vi "ControlInterface.vi"() -> ()   [LabVIEW 2016]
uses:
  Classes/CAlex2-Display/CAlex2_Display.lvclass
  D:/JinXin/LabVIEW.git/CAlex2-Controller-treadmill/Classes/SerialChain/SerialChain.lvclass
  D:/JinXin/LabVIEW.git/CAlex2-Controller-treadmill/Classes/CAlex2/CAlex2.lvclass
  Classes/ForceField/TypeDef/FF_Gains.ctl
  Classes/CAlex2/TypeDef/LowerBodyDim.ctl
  Classes/MotorControl/TypeDef/ControllerMode.ctl
  Classes/MotorControl/MotorControl.lvclass
  Classes/CAlex2/CAlex2.lvclass
  Classes/SerialChain/SerialChain.lvclass
  Classes/ForceField/ForceField.lvclass
  <vilib>/GoldZinc Software/auzn custom VIs/CustomVI.lvlib
panel:
  in  "FF Disp Type":enum16{"FF: XYZ", "FF: NTD"}(ring)
  in  "Motor Mode":T1={"Idle"=FALSE, "Pre"=FALSE, "Pre-Value"=7, "PID"=FALSE} {"Pre-Value" items=["7N"=7, "10N"=10, "15N"=15, "20N"=20]}
  out "ViconConnected":bool
  in  "ResetIMU":bool
  in  "Vicon":bool
  in  "Extra Wt":cluster{"Thigh (lb)":dbl, "Shank (lb)":dbl}
  in  "UpdateFF":bool
  in  "XZ":bool
  in  "YZ":bool
  in  "XY":bool
  out "R_Hill":u32(colorbox)
  out "R_Ball":u32(colorbox)
  out "R_Toe":u32(colorbox)
  out "L_Hill":u32(colorbox)
  out "L_Ball":u32(colorbox)
  out "L_Toe":u32(colorbox)
  in  "Status 8":bool
  out "Waveform Chart 8":cluster{"[0]":dbl, "[1]":dbl}(graph)
  in  "Cuff Location":T2={"Hip Wd (m)"=0.42, "Hip Ht (m)"=0.2, "ThighDist (in)"=1.5, "ThighToKnee"=0.1, "Hip Fwd (m)"=-0.02, "ShankToKnee"=0.1}
  in  "Force Field":bool
  in  "LegWeight":bool
  in  "CuffWeight":bool
  out "Normal Force Shape":cluster{dbl[], dbl[]}[](graph)
  in  "File Name":string
  out "Record Time":dbl format="%.2f"
  in  "Leg Property":T3={"Thigh"=0.42, "Shank"=0.42, "ShankWt"=0.0, "ThighWt"=0.0, "Hip"=0.32}
  in  "Gains":T4
  in  "Reset":bool
  in  "Stop RT":bool
  in  "Status 7":bool
  in  "Status 6":bool
  in  "Status 5":bool
  in  "Status 4":bool
  in  "Status 3":bool
  in  "Status 2":bool
  in  "Status 1":bool
  out "Waveform Chart 7":cluster{"[0]":dbl, "[1]":dbl}(graph)
  out "Waveform Chart 6":cluster{"[0]":dbl, "[1]":dbl}(graph)
  out "Waveform Chart 5":cluster{"[0]":dbl, "[1]":dbl}(graph)
  out "Waveform Chart 4":cluster{"[0]":dbl, "[1]":dbl}(graph)
  out "Waveform Chart 3":cluster{"[0]":dbl, "[1]":dbl}(graph)
  out "Waveform Chart 2":cluster{"[0]":dbl, "[1]":dbl}(graph)
  out "Waveform Chart 1":cluster{"[0]":dbl, "[1]":dbl}(graph)
  in  "ZeroPosition":bool
  in  "Force Field Type":u8(ring)=1 items=["Ankle Traj", "Ankle Traj 2", "No FF", "Ankle Traj Old"]
  in  "Record Data?":bool
  out "Planned Tensions":dbl[](array[numeric]) format="%.2f"
  out "Motor Command":dbl[](array[numeric]) format="%.5f"
  out "Ankle Center":dbl[](array[numeric]) format="%.4f"
  out "Force Field":dbl[](array[numeric]) format="%.2f"
  out "Joint Angles":dbl[](array[numeric]) format="%.1f"
  in  "TareIMU":bool
  in  "Leg Position":refnum<k7>(container)
  # "C-ALEX Control Interface V2 \nDeveloped by Xin Jin, ROAR Laboratory, Columbia University"
  # "Leg Pose"
  # "Status Monitor"
  # "Data Record"
  # "Subject Information"
  # "Foot Switches"
  # "Force Field"
  # "Control Panel"
  # "Motor Mode"
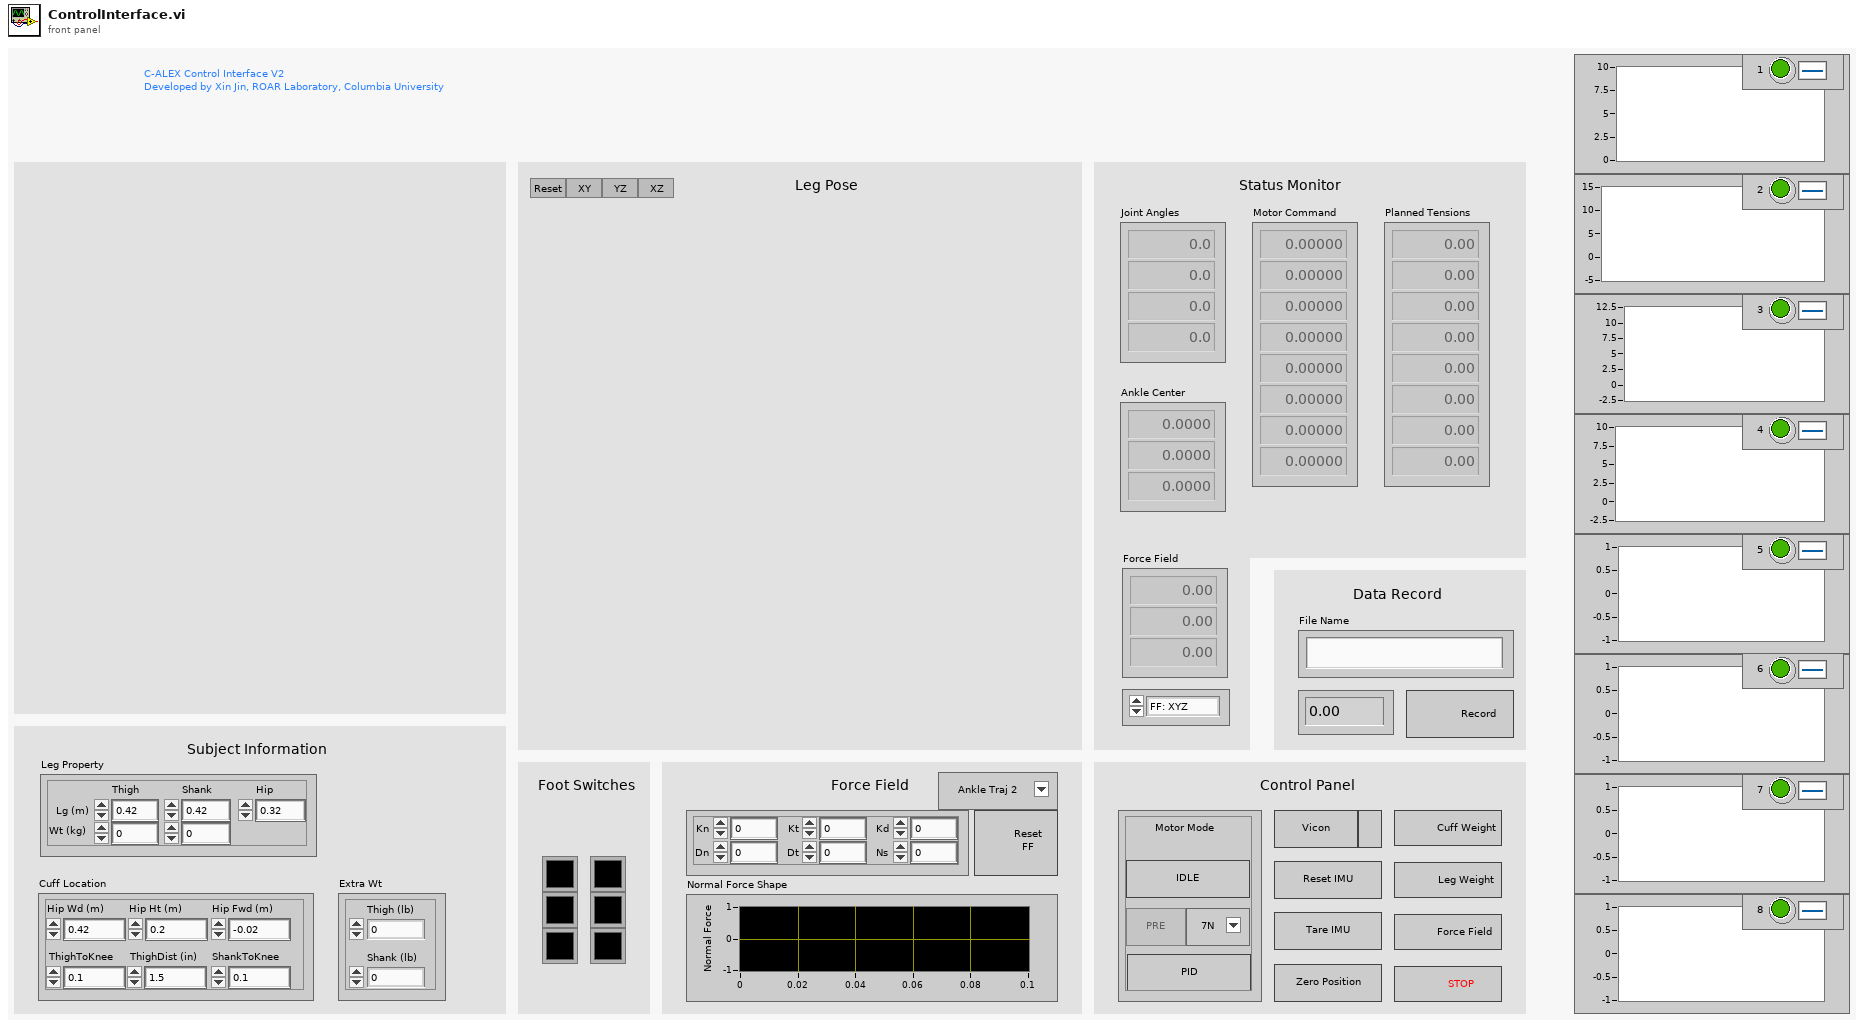
[diagram p1: front panel]
types:
  T1 = cluster{"Idle":bool, "Pre":bool, "Pre-Value":u8, "PID":bool}
  T2 = cluster{"Hip Wd (m)":dbl, "Hip Ht (m)":dbl, "ThighDist (in)":dbl, "ThighToKnee":dbl, "Hip Fwd (m)":dbl, "ShankToKnee":dbl}
  T3 = cluster{"Thigh":dbl, "Shank":dbl, "ShankWt":dbl, "ThighWt":dbl, "Hip":dbl}
  T4 = cluster{"Kn":dbl, "Dn":dbl, "Kt":dbl, "Dt":dbl, "Kd":dbl, "Ns":dbl}
  T5 = cluster{"AxisLabel":string[], "AxisMax":dbl[], "AxisMin":dbl[]}
  T6 = typedef "ForceField.lvclass/FF_Gains.ctl" = cluster{"Kn":dbl, "Dn":dbl, "Kt":dbl, "Dt":dbl, "Kd":dbl, "Ns":dbl}
  T7 = typedef "CAlex2.lvclass/LowerBodyDim.ctl" = cluster{"BodyDim":cluster{"ThighLt (m)":dbl, "ShankLt (m)":dbl, "HipWd (m)":dbl}, "BodyWt":cluster{"Thigh (kg)":dbl, "Shank (kg)":dbl}, "Cuff Loc":cluster{"HipCuffWd (m)":dbl, "HipCuffHt (m)":dbl, "HipFwdShift (m)":dbl, "ThighToKnee (m)":dbl, "ThighCuffDist (m)":dbl, "ShankToKnee (m)":dbl}}
  T8 = typedef "MotorControl.lvclass/ControllerMode.ctl" = enum16{"Idle", "FF", "PID"}
  T9 = enum8{"Enabled", "Disabled", "Disabled and Grayed Out"}
  T10 = cluster{"Input":enum16{"Fr:Cable", "Fr:Motor", "Fr:Sensor"}, "Output":enum16{"To:Cable", "To:Motor", "To:Sensor"}}
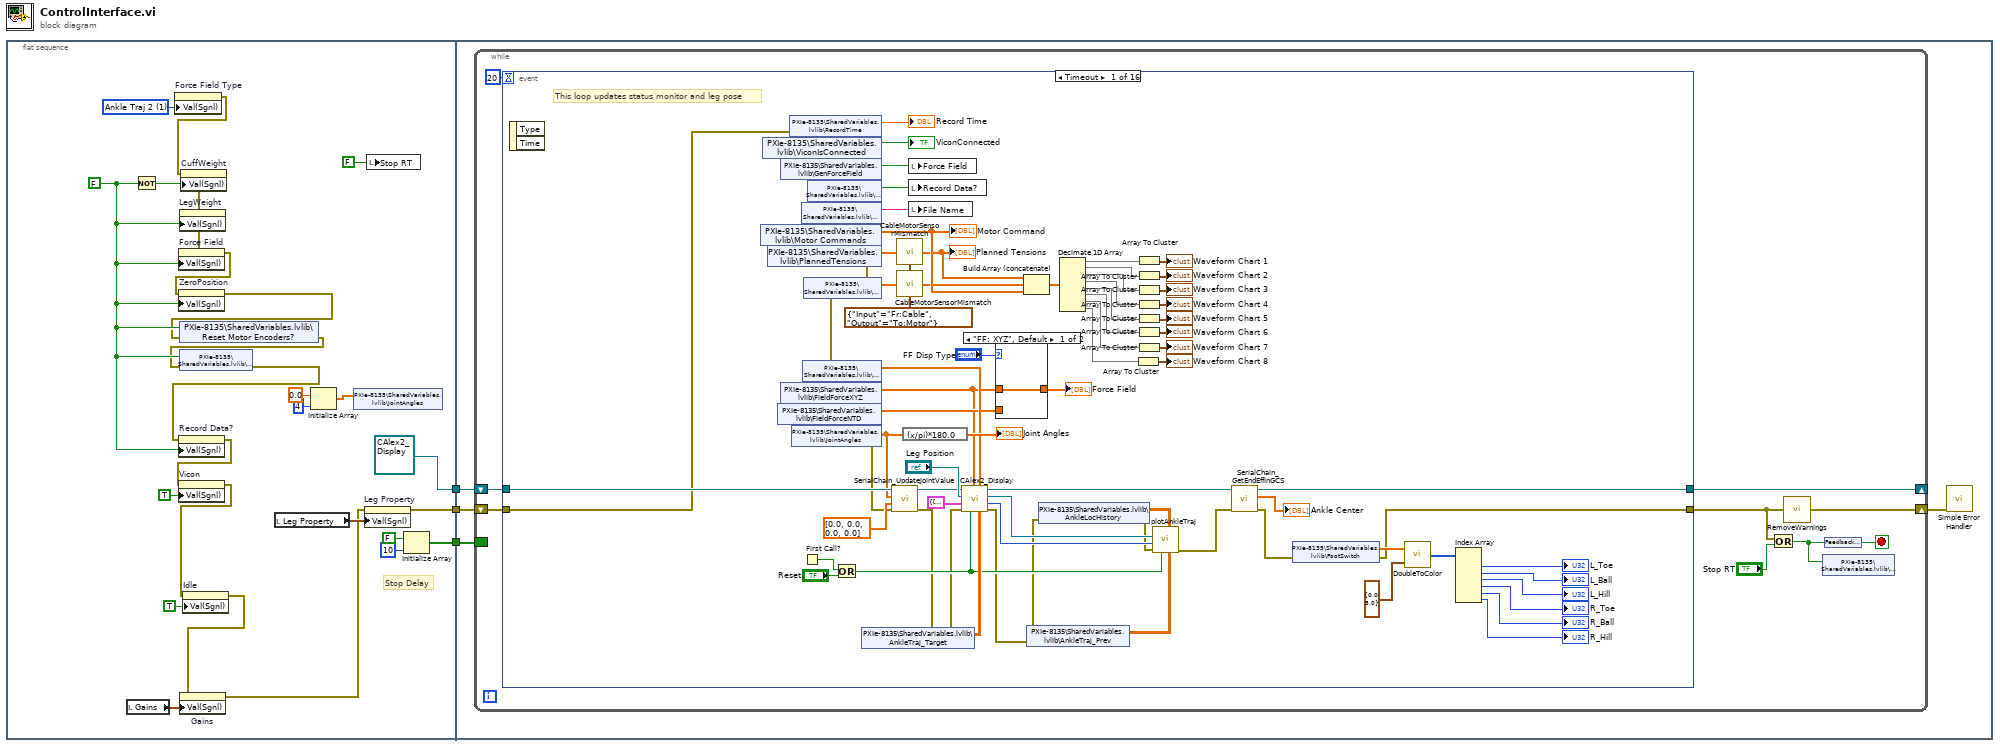
[diagram p0: block diagram]
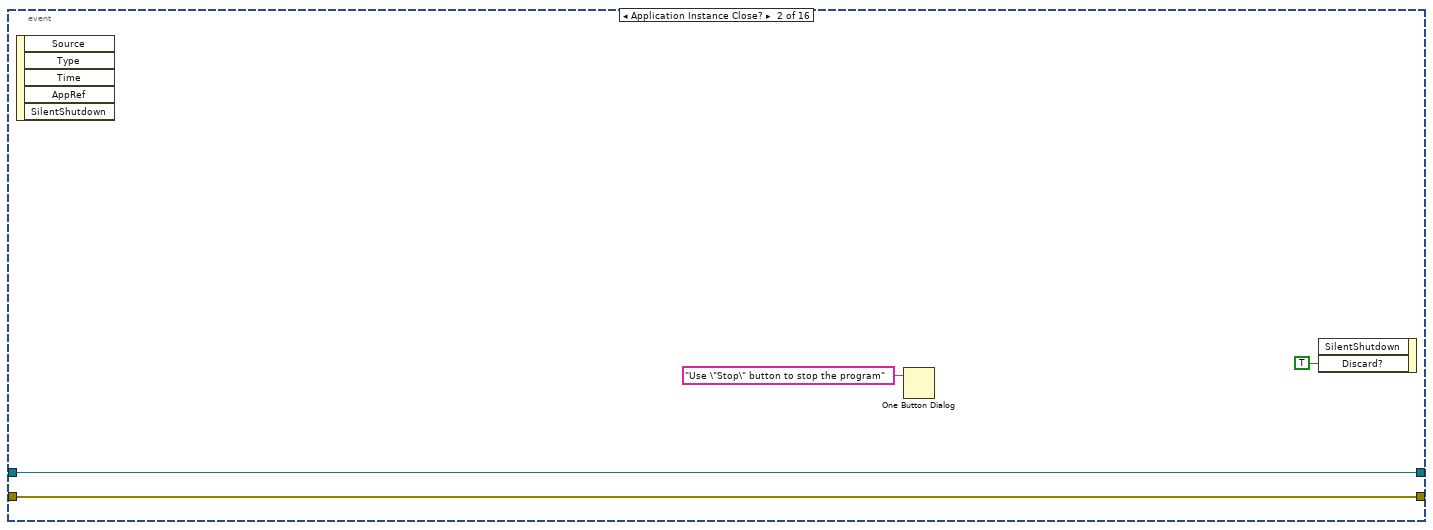
[diagram p3: hidden frame]
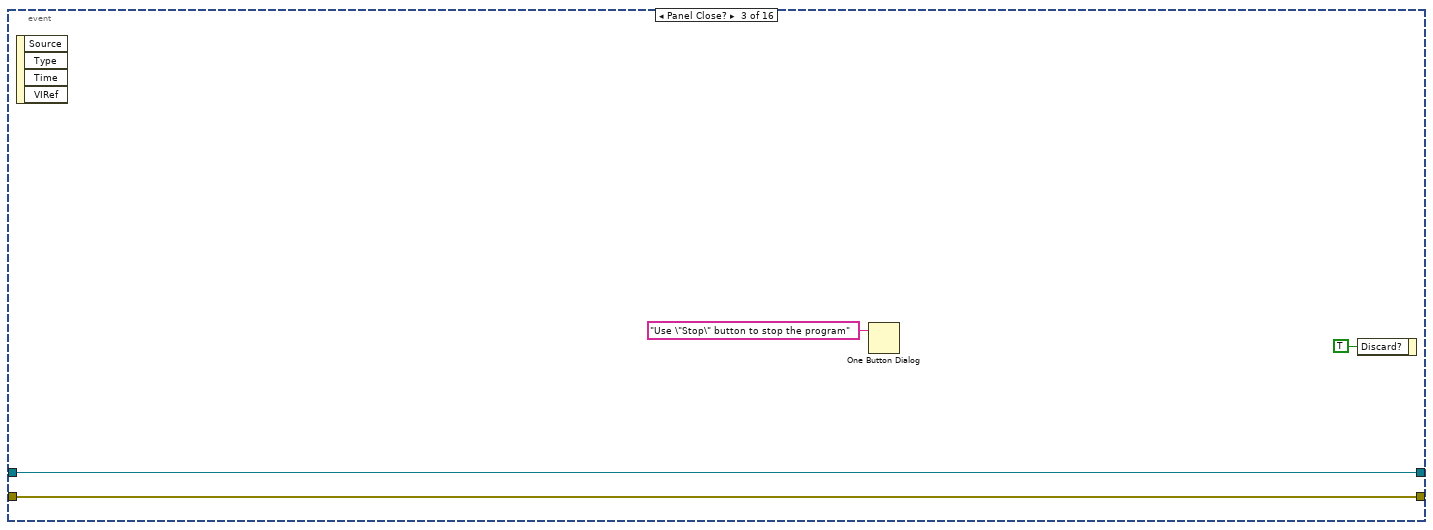
[diagram p4: hidden frame]
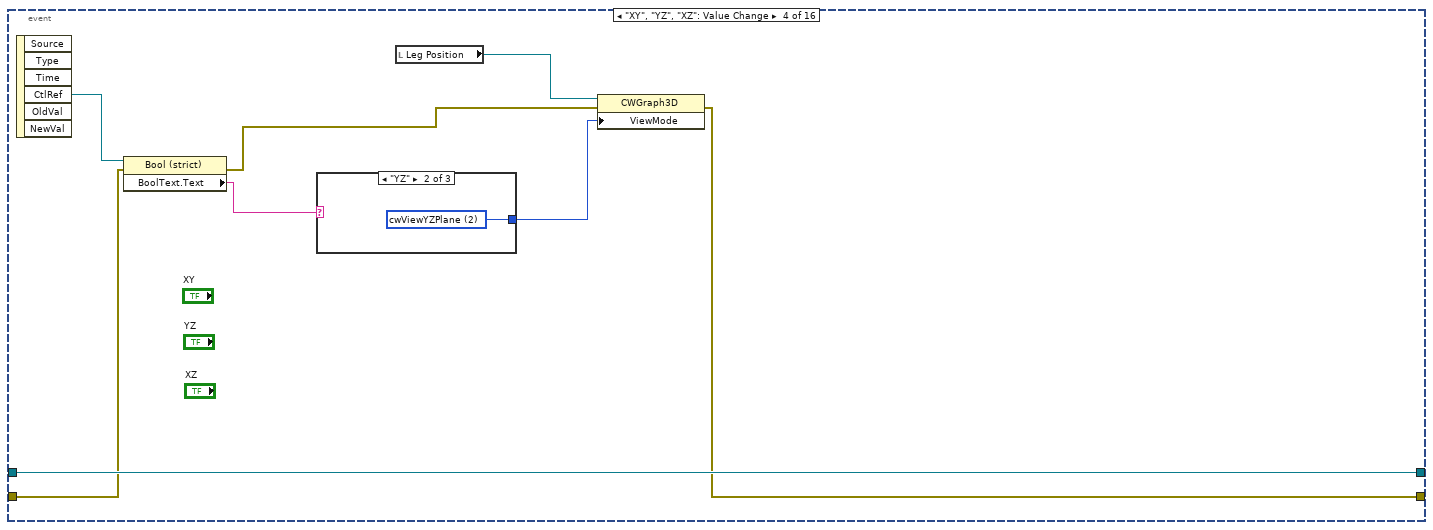
[diagram p5: hidden frame]
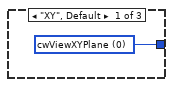
[diagram p6: hidden frame]
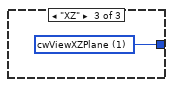
[diagram p7: hidden frame]
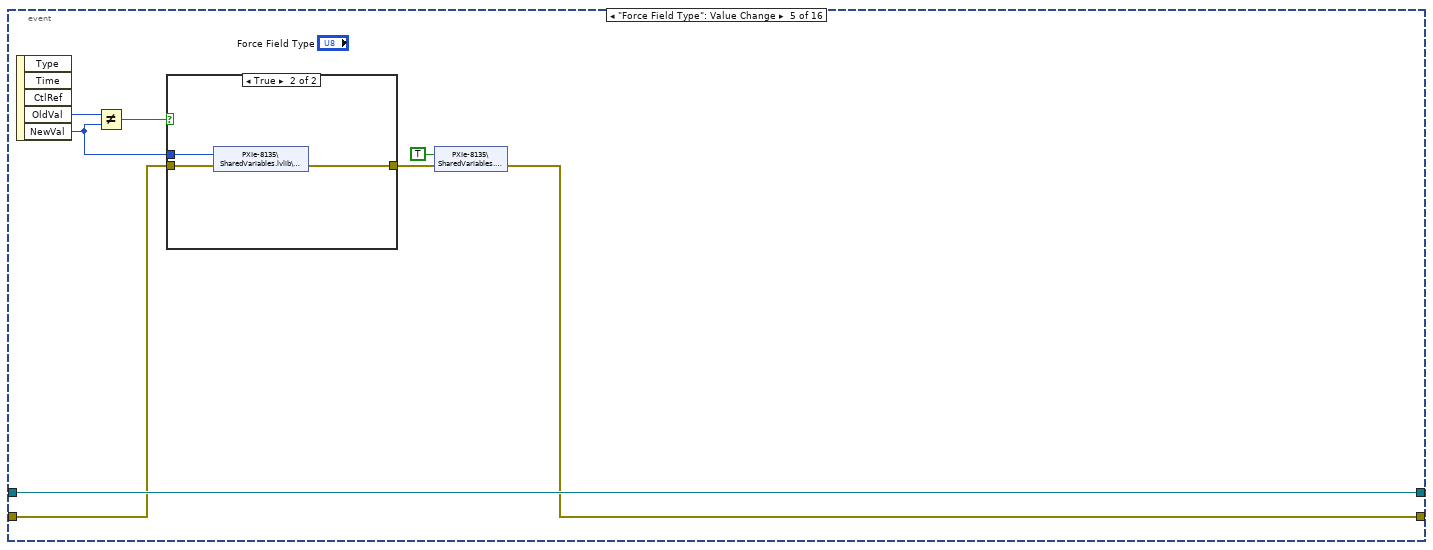
[diagram p8: hidden frame]
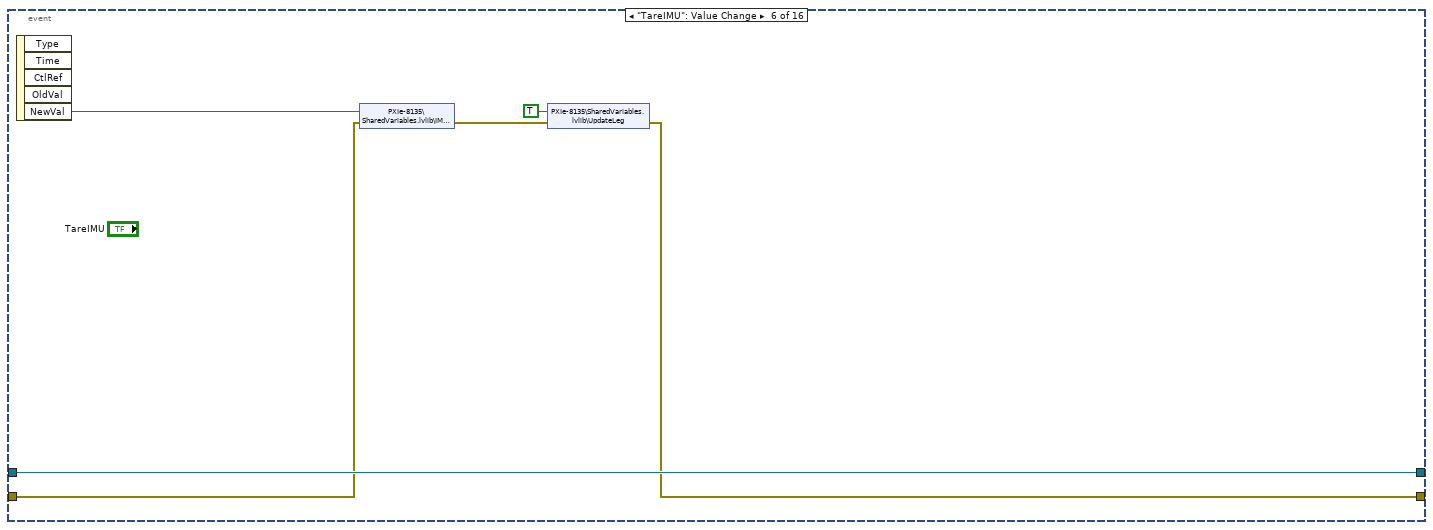
[diagram p10: hidden frame]
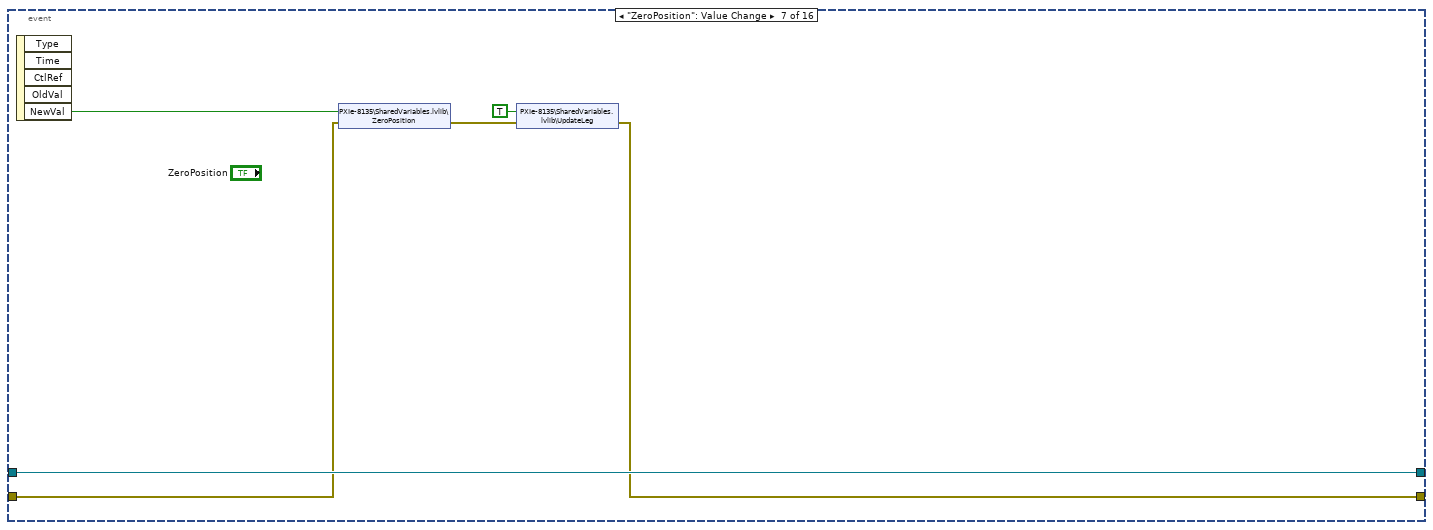
[diagram p11: hidden frame]
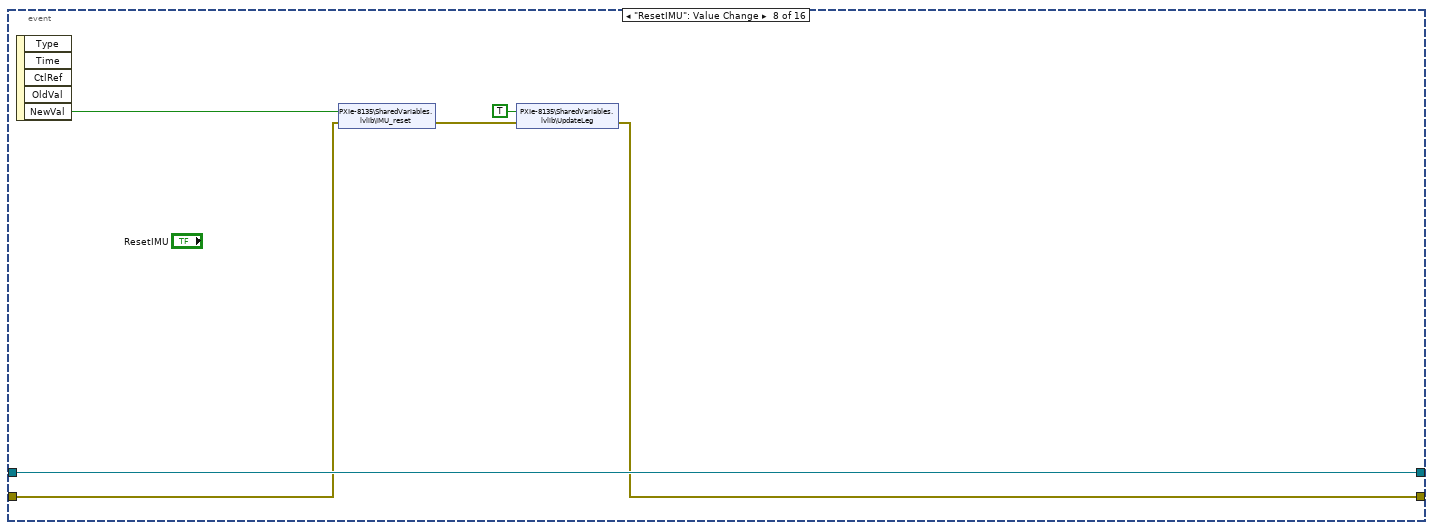
[diagram p12: hidden frame]
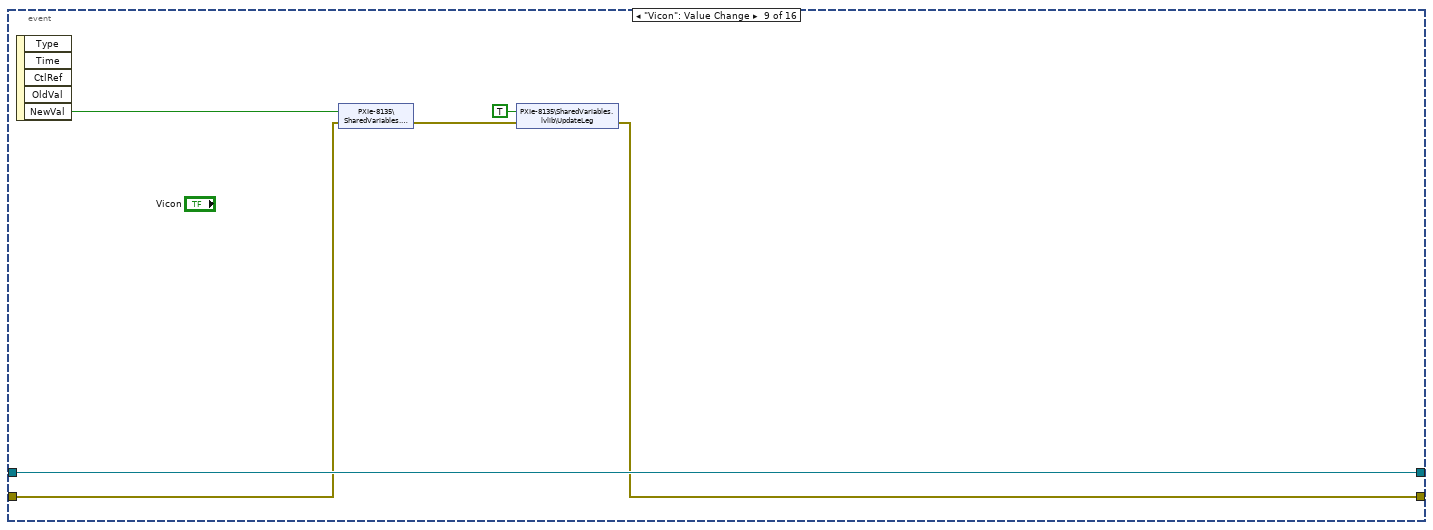
[diagram p13: hidden frame]
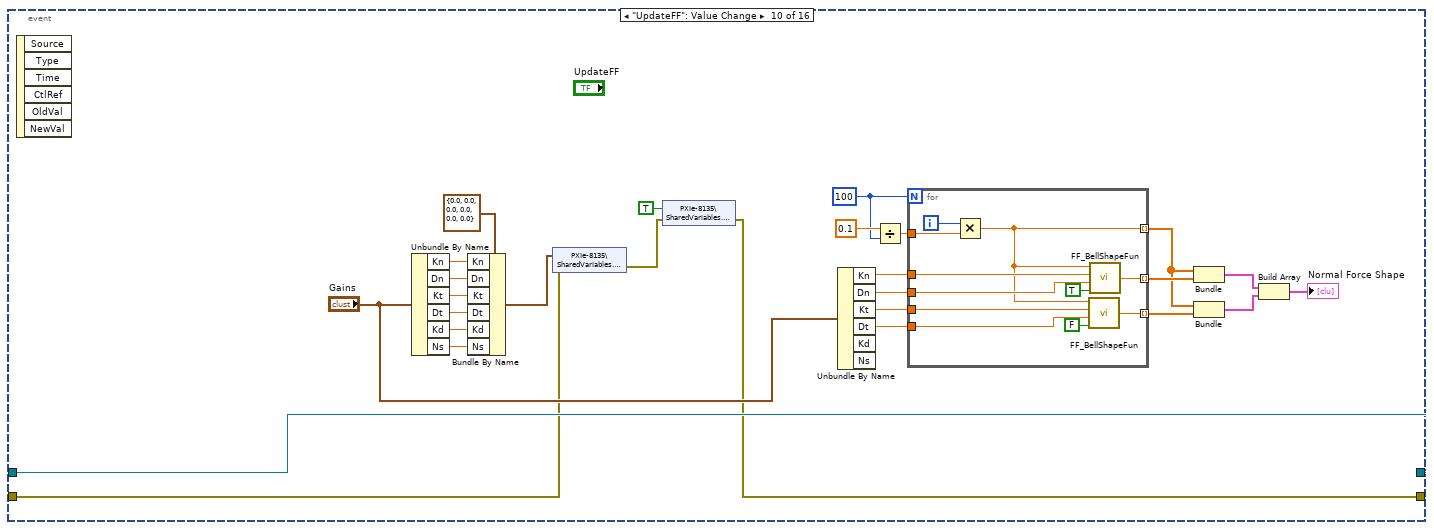
[diagram p14: hidden frame]
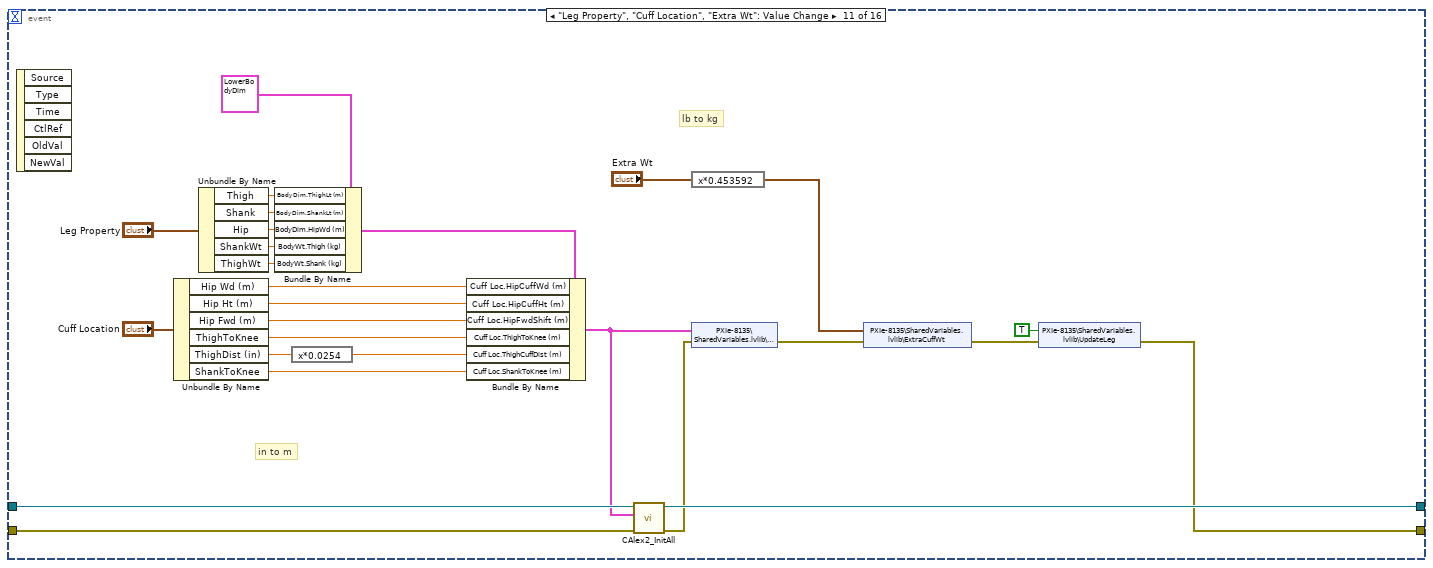
[diagram p15: hidden frame]
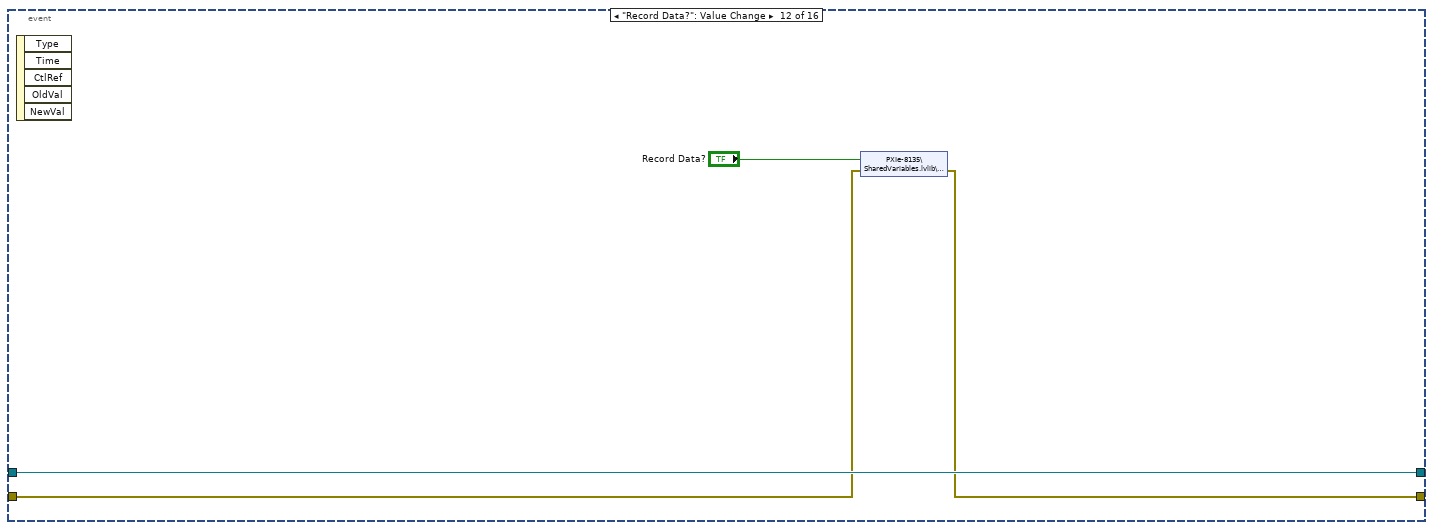
[diagram p16: hidden frame]
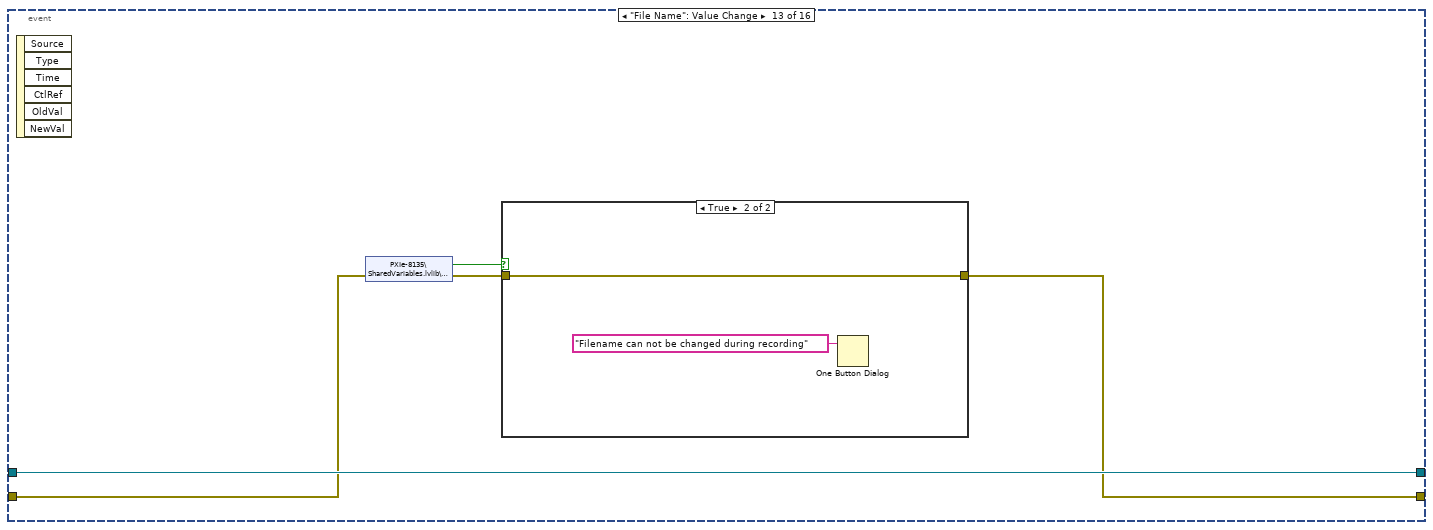
[diagram p17: hidden frame]
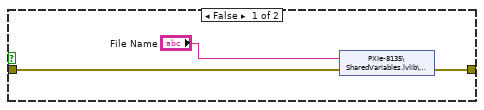
[diagram p18: hidden frame]
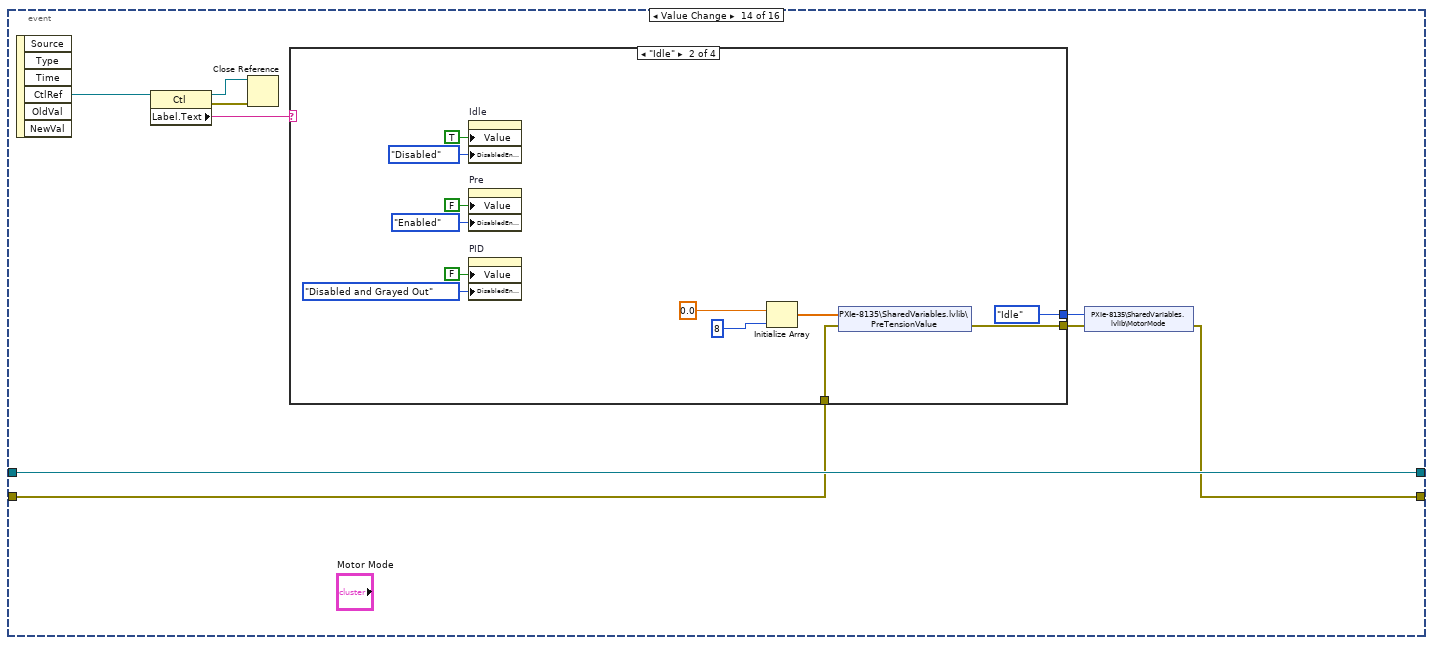
[diagram p19: hidden frame]
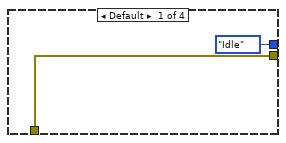
[diagram p20: hidden frame]
diagram:
  n1 = flat-sequence {
    tunnel: [w28] -> w3
    tunnel: [refnum<class "CAlex2_Display.lvclass"> refnum ("CAlex2")] -> w2
    tunnel: [w22] -> w1
    tunnel: w3 -> [w32]
    tunnel: w2 -> [w34]
    tunnel: w1 -> [w33]
    frame #0 {
      w17 = u8 1 items=["Ankle Traj", "Ankle Traj 2", "No FF", "Ankle Traj Old"] ("Force Field Type")
      w10 = FALSE ("Es SH Center?")
      # "Stop Delay"
      n2 = local read "Gains"() -> (w27:T4)
      n3 = Not(x=w10) -> (.not. x?=w11:bool)
      n4 = property on="Force Field Type" class="Ring (strict)"("Val(Sgnl)"=w17) -> (error out=w5:errorcluster)  [unwired: 2 in, 1 out]
      n5 = property on="CuffWeight" class="Bool (strict)"(error in=w5, "Val(Sgnl)"=w11) -> (error out=w13:errorcluster)  [unwired: 1 in, 1 out]
      n6 = property on="LegWeight" class="Bool (strict)"(error in=w13, "Val(Sgnl)"=w10) -> (error out=w12:errorcluster)  [unwired: 1 in, 1 out]
      n7 = property on="Force Field" class="Bool (strict)"(error in=w12, "Val(Sgnl)"=w10) -> (error out=w9:errorcluster)  [unwired: 1 in, 1 out]
      n8 = property on="ZeroPosition" class="Bool (strict)"(error in=w9, "Val(Sgnl)"=w10) -> (error out=w8:errorcluster)  [unwired: 1 in, 1 out]
      n9 = shared-variable "PXIe-8135\\SharedVariables.lvlib\\Reset Motor Encoders?"(w10, error in=w8) -> (error out=w7:errorcluster)
      n10 = shared-variable "PXIe-8135\\SharedVariables.lvlib\\Stop RT"(w10, error in=w7) -> (error out=w4:errorcluster)
      n11 = property on="Record Data?" class="Bool (strict)"(error in=w4, "Val(Sgnl)"=w10) -> (error out=w15:errorcluster)  [unwired: 1 in, 1 out]
      n12 = property on="Vicon" class="Bool (strict)"(error in=w15, "Val(Sgnl)"=TRUE ("Value (Signaling)")) -> (error out=w16:errorcluster)  [unwired: 1 in, 1 out]
      n13 = property on="Idle" class="Bool (strict)"(error in=w16, "Val(Sgnl)"=TRUE ("Value")) -> (error out=w6:errorcluster)  [unwired: 1 in, 1 out]
      n14 = property on="Gains" class="Clust (strict)"(error in=w6, "Val(Sgnl)"=w27) -> (error out=w26:errorcluster)  [unwired: 1 in, 1 out]
      n15 = local read "Leg Property"() -> (w29:T3)
      n16 = Initialize Array(0.0 ("element"), 4 ("dimension size")) -> (w20:dbl[])
      n17 = shared-variable "PXIe-8135\\SharedVariables.lvlib\\JointAngles"(w20) -> ()  [unwired: 1 in, 1 out]
      n18 = property on="Leg Property" class="Clust (strict)"(error in=w26, "Val(Sgnl)"=w29) -> (error out=w28:errorcluster)  [unwired: 1 in, 1 out]
      n19 = local write "Stop RT"(FALSE ("Es SH Center?")) -> ()
      n20 = Initialize Array(FALSE, 10 ("dimension size")) -> (w22:bool[])
    }
    frame #1 {
      n21 = while {
        shift-right: [w41] -> _
        shift-left: w34 -> [w42]
        border: w33 -> [_]
        shift-right: [w38] -> w31
        shift-left: w32 -> [w39]
        stop <- w40 stop-if-true
        n22 = event shown="[0] Timeout" {
          selector: _ -> [_ _ _ _ _ _ _ _ _ _ _ _ _ _ _ _]
          dyn-events: _ -> [_ _ _ _ _ _ _ _ _ _ _ _ _ _ _ _]
          timeout: 20 -> [_ _ _ _ _ _ _ _ _ _ _ _ _ _ _ _]
          tunnel: [w70 w130 w134 w139 w148 w160 w167 w173 w179 w182 w241 w248 w254 w263 w306 w314] -> w37
          tunnel: w42 -> [w106 w129 w133 w142 w150 w163 w169 w175 w181 w208 w246 w250 w255 w269 w312 w324]
          tunnel: w39 -> [w44 w130 w134 w136 w147 w161 w168 w174 w180 w183 w244 w247 w253 w261 w305 w315]
          tunnel: [w104 w129 w133 w142 w150 w163 w169 w175 w181 w208 w245 w250 w255 w269 w312 w324] -> w41
          event Timeout {
            w71 = T10 {"Input"=enum."Fr:Cable", "Output"=enum."To:Motor"} ("Conversion")
            # "This loop updates status monitor and leg pose"
            n23 = event-data() -> ()  [unwired: 1 in, 2 out]
            n24 = shared-variable "PXIe-8135\\SharedVariables.lvlib\\RecordTime"(error in=w44) -> (→"Record Time":dbl, error out=w76:errorcluster)
            n25 = shared-variable "PXIe-8135\\SharedVariables.lvlib\\ViconIsConnected"(error in=w76) -> (→"ViconConnected":bool, error out=w52:errorcluster)
            n26 = shared-variable "PXIe-8135\\SharedVariables.lvlib\\GenForceField"(error in=w52) -> (w61:bool, error out=w62:errorcluster)
            n27 = First Call?() -> (First Call?: T/F=w107:bool)
            n28 = shared-variable "PXIe-8135\\SharedVariables.lvlib\\Record?"(error in=w62) -> (w59:bool, error out=w60:errorcluster)
            n29 = shared-variable "PXIe-8135\\SharedVariables.lvlib\\FileName"(error in=w60) -> (w51:string, error out=w50:errorcluster)
            n30 = shared-variable "PXIe-8135\\SharedVariables.lvlib\\Motor Commands"(error in=w50) -> (w100:dbl[], error out=w124:errorcluster)
            "Motor Command" <- w100
            n31 = shared-variable "PXIe-8135\\SharedVariables.lvlib\\PlannedTensions"(error in=w124) -> (w73:dbl[], error out=w101:errorcluster)
            n32 = shared-variable "PXIe-8135\\SharedVariables.lvlib\\Tensions"(error in=w101) -> (w75:dbl[], error out=w45:errorcluster)
            n33 = shared-variable "PXIe-8135\\SharedVariables.lvlib\\ClosestPt"(error in=w45) -> (w92:dbl[], error out=w69:errorcluster)
            n34 = shared-variable "PXIe-8135\\SharedVariables.lvlib\\FieldForceXYZ"(error in=w69) -> (w55:dbl[], error out=w53:errorcluster)
            n35 = shared-variable "PXIe-8135\\SharedVariables.lvlib\\FieldForceNTD"(error in=w53) -> (w56:dbl[], error out=w47:errorcluster)
            n36 = shared-variable "PXIe-8135\\SharedVariables.lvlib\\JointAngles"(error in=w47) -> (w102:dbl[], error out=w46:errorcluster)
            n37 = Or(x=w107, y="Reset") -> (x .or. y?=w89:bool)
            n38 = call "SerialChain_UpdateJointValue.vi"("error in (no error)"=w46, "JointSpeed (rad/s | m/s)"=dbl[] [0.0, 0.0, 0.0, 0.0] ("JointSpeed (rad)"), "JointAngle (rad | m)"=w102, "SerialChain in"=w106) -> ("error out"=w48:errorcluster, "SerialChain out"=w96:refnum<class "CAlex2_Display.lvclass">)  [unwired: 6 in]
            n39 = shared-variable "PXIe-8135\\SharedVariables.lvlib\\AnkleTraj_Target"(error in=w48) -> (w93:dbl[][], error out=w68:errorcluster)
            n40 = call "CableMotorSensorMismatch.vi"("Conversion"=w71, "Input"=w73) -> ("Output"=w72:dbl[])  [unwired: 2 in]
            "Planned Tensions" <- w72
            n41 = call "CableMotorSensorMismatch.vi"("Conversion"=w71, "Input"=w75) -> ("Output"=w74:dbl[])  [unwired: 2 in]
            n42 = expression code="(x/pi)*180.0" ("radians to degrees")(w102) -> (→"Joint Angles":dbl[])
            n43 = local write "Force Field"(w61) -> ()
            n44 = local write "Record Data?"(w59) -> ()
            n45 = local write "File Name"(w51) -> ()
            n46 = call "CAlex2_Display.vi"("AnkleTraj_Target"=w93, "ClosePt"=w92, "Init?"=w89, "Field Force"=w55, "error in (no error)"=w68, "AxisSetting"=T5 {"AxisLabel"=["x ", "y", "z "], "AxisMax"=[0.75, 0.3, 0.8], "AxisMin"=[-0.75, -1.2, -0.7]}, "3D graph in"="Leg Position", "CLX2 in"=w96) -> ("error out"=w67:errorcluster, "LastPlotNum"=w90:i32, "3D graph out"=w91:refnum<k7>, "CLX2 out"=w98:refnum<class "CAlex2_Display.lvclass">)
            n47 = case shown="\"FF: XYZ\", Default" "FF Disp Type" {
              tunnel: w56 -> [_ w126]
              tunnel: w55 -> [w125 _]
              tunnel: [w125 w126] -> w54
              frame "FF: XYZ", Default {
              }
              frame "FF: NTD" {
              }
            }
            "Force Field" <- w54
            n48 = Build Array (concatenate)(w72, w74, w100) -> (w99:dbl[])
            n49 = shared-variable "PXIe-8135\\SharedVariables.lvlib\\AnkleTraj_Prev"(error in=w67) -> (w88:dbl[][], error out=w64:errorcluster)
            n50 = shared-variable "PXIe-8135\\SharedVariables.lvlib\\AnkleLocHistory"(error in=w64) -> (w65:dbl[][], error out=w63:errorcluster)
            n51 = Decimate 1D Array(w99) -> (w117:dbl[], w116:dbl[], w122:dbl[], w121:dbl[], w120:dbl[], w119:dbl[], w118:dbl[], w49:dbl[])
            n52 = Array To Cluster(array=w49) -> (cluster=→"Waveform Chart 8":cluster{"[0]":dbl, "[1]":dbl})
            n53 = Array To Cluster(array=w117) -> (cluster=→"Waveform Chart 1":cluster{"[0]":dbl, "[1]":dbl})
            n54 = Array To Cluster(array=w116) -> (cluster=→"Waveform Chart 2":cluster{"[0]":dbl, "[1]":dbl})
            n55 = Array To Cluster(array=w122) -> (cluster=→"Waveform Chart 3":cluster{"[0]":dbl, "[1]":dbl})
            n56 = Array To Cluster(array=w121) -> (cluster=→"Waveform Chart 4":cluster{"[0]":dbl, "[1]":dbl})
            n57 = Array To Cluster(array=w120) -> (cluster=→"Waveform Chart 5":cluster{"[0]":dbl, "[1]":dbl})
            n58 = Array To Cluster(array=w119) -> (cluster=→"Waveform Chart 6":cluster{"[0]":dbl, "[1]":dbl})
            n59 = Array To Cluster(array=w118) -> (cluster=→"Waveform Chart 7":cluster{"[0]":dbl, "[1]":dbl})
            n60 = call "plotAnkleTraj.vi"("AnkleTraj_Prev"=w88, "AnkleTraj_history"=w65, "Init?"=w89, "error in (no error)"=w63, "PreviousPlotNum"=w90, "3D graph in"=w91) -> ("error out"=w66:errorcluster)  [unwired: 3 in, 2 out]
            n61 = call "SerialChain_GetEndEffInGCS.vi"("error in (no error)"=w66, "SerialChain in"=w98) -> ("error out"=w58:errorcluster, "Pendeff(GCS)"=→"Ankle Center":dbl[], "SerialChain out"=w104:refnum<class "CAlex2_Display.lvclass">)  [unwired: 5 in, 2 out]
            n62 = shared-variable "PXIe-8135\\SharedVariables.lvlib\\FootSwitch"(error in=w58) -> (w87:dbl[], error out=w70:errorcluster)
            n63 = call <vilib>:"DoubleToColor.vi"("Value Range"=cluster{"ValueMin":dbl, "ValueMax":dbl} {"ValueMin"=0.0, "ValueMax"=5.0}, "Data"=w87) -> ("Colors"=w85:u32[])  [unwired: 1 in]
            n64 = Index Array(array=w85) -> (element #1=→"L_Toe":u32, element #2=→"L_Ball":u32, element #3=→"L_Hill":u32, element #4=→"R_Toe":u32, element #5=→"R_Ball":u32, element #6=→"R_Hill":u32)  [unwired: 6 in]
          }
          event Application Instance Close? {
            n65 = event-data() -> ()  [unwired: 1 in, 5 out]
            n66 = One Button Dialog(message="Use \"Stop\" button to stop the program") -> ()  [unwired: 1 in, 1 out]
            n67 = event-data("Discard?"=TRUE) -> ()  [unwired: 2 in, 1 out]
          }
          event Panel Close? {
            n68 = event-data() -> ()  [unwired: 1 in, 4 out]
            n69 = One Button Dialog(message="Use \"Stop\" button to stop the program") -> ()  [unwired: 1 in, 1 out]
            n70 = event-data("Discard?"=TRUE) -> ()  [unwired: 1 in, 1 out]
          }
          event "XY", "YZ", "XZ": Value Change {
            n71 = event-data() -> ("CtlRef"=w138:refnum<vi>)  [unwired: 1 in, 5 out]
            n72 = property class="Bool (strict)"(reference=w138, error in=w136) -> (error out=w137:errorcluster, "BoolText.Text"=w135:string)  [unwired: 1 out]
            n73 = case shown="\"YZ\"" w135 {
              tunnel: [w143 w144 w145] -> w140
              frame "XY", Default {
                w143 = 0 items=["cwViewXYPlane", "cwViewXZPlane", "cwViewYZPlane", "cwViewUserDefined"] ("ViewMode")
              }
              frame "YZ" {
                w144 = 2 items=["cwViewXYPlane", "cwViewXZPlane", "cwViewYZPlane", "cwViewUserDefined"] ("ViewMode")
              }
              frame "XZ" {
                w145 = 1 items=["cwViewXYPlane", "cwViewXZPlane", "cwViewYZPlane", "cwViewUserDefined"] ("ViewMode")
              }
            }
            n74 = local read "Leg Position"() -> (w141:refnum<k7>)
            n75 = property class="CWGraph3D"(reference=w141, error in=w137, "ViewMode"=w140) -> (error out=w139:errorcluster)  [unwired: 1 out]
          }
          event "Force Field Type": Value Change {
            n76 = event-data() -> ("OldVal"=w153:u8, "NewVal"=w151:u8)  [unwired: 1 in, 3 out]
            n77 = Not Equal?(x=w153, y=w151) -> (x != y?=w152:bool)
            n78 = case shown="True" w152 {
              tunnel: w151 -> [_ w157]
              tunnel: [w154 w155] -> w149
              tunnel: w147 -> [w154 w156]
              frame False {
              }
              frame True {
                n79 = shared-variable "PXIe-8135\\SharedVariables.lvlib\\PathType"(w157, error in=w156) -> (error out=w155:errorcluster)
              }
            }
            n80 = shared-variable "PXIe-8135\\SharedVariables.lvlib\\FFRst"(TRUE ("UpdateArm"), error in=w149) -> (error out=w148:errorcluster)
          }
          event "TareIMU": Value Change {
            n81 = event-data() -> ("NewVal"=w162:bool)  [unwired: 1 in, 4 out]
            n82 = shared-variable "PXIe-8135\\SharedVariables.lvlib\\IMU_Tare"(w162, error in=w161) -> (error out=w158:errorcluster)
            n83 = shared-variable "PXIe-8135\\SharedVariables.lvlib\\UpdateLeg"(TRUE ("UpdateArm"), error in=w158) -> (error out=w160:errorcluster)
          }
          event "ZeroPosition": Value Change {
            n84 = event-data() -> ("NewVal"=w166:bool)  [unwired: 1 in, 4 out]
            n85 = shared-variable "PXIe-8135\\SharedVariables.lvlib\\ZeroPosition"(w166, error in=w168) -> (error out=w164:errorcluster)
            n86 = shared-variable "PXIe-8135\\SharedVariables.lvlib\\UpdateLeg"(TRUE ("UpdateArm"), error in=w164) -> (error out=w167:errorcluster)
          }
          event "ResetIMU": Value Change {
            n87 = event-data() -> ("NewVal"=w172:bool)  [unwired: 1 in, 4 out]
            n88 = shared-variable "PXIe-8135\\SharedVariables.lvlib\\IMU_reset"(w172, error in=w174) -> (error out=w170:errorcluster)
            n89 = shared-variable "PXIe-8135\\SharedVariables.lvlib\\UpdateLeg"(TRUE ("UpdateArm"), error in=w170) -> (error out=w173:errorcluster)
          }
          event "Vicon": Value Change {
            n90 = event-data() -> ("NewVal"=w178:bool)  [unwired: 1 in, 4 out]
            n91 = shared-variable "PXIe-8135\\SharedVariables.lvlib\\Vicon"(w178, error in=w180) -> (error out=w176:errorcluster)
            n92 = shared-variable "PXIe-8135\\SharedVariables.lvlib\\UpdateLeg"(TRUE ("UpdateArm"), error in=w176) -> (error out=w179:errorcluster)
          }
          event "UpdateFF": Value Change {
            w193 = 100
            n93 = event-data() -> ()  [unwired: 1 in, 6 out]
            n94 = Unbundle By Name("Gains") -> ("Kn"=w207:dbl, "Dn"=w205:dbl, "Kt"=w204:dbl, "Dt"=w203:dbl, "Kd"=w202:dbl, "Ns"=w201:dbl)
            n95 = Bundle By Name(cluster=T6 {"Kn"=0.0, "Dn"=0.0, "Kt"=0.0, "Dt"=0.0, "Kd"=0.0, "Ns"=0.0} ("Gains"), "Kn"=w207, "Dn"=w205, "Kt"=w204, "Dt"=w203, "Kd"=w202, "Ns"=w201) -> (w200:T6)
            n96 = shared-variable "PXIe-8135\\SharedVariables.lvlib\\Gains"(w200, error in=w183) -> (error out=w184:errorcluster)
            n97 = shared-variable "PXIe-8135\\SharedVariables.lvlib\\FFRst"(TRUE ("UpdateArm"), error in=w184) -> (error out=w182:errorcluster)
            n98 = Unbundle By Name("Gains") -> ("Kn"=w198:dbl, "Dn"=w197:dbl, "Kt"=w196:dbl, "Dt"=w195:dbl)  [unwired: 2 out]
            n99 = Divide(x=0.1, y=w193) -> (x/y=w192:dbl)
            n100 = for {
              N: w193 -> [_]
              tunnel: w198 -> [w219]
              tunnel: w197 -> [w218]
              tunnel: w196 -> [w217]
              tunnel: w195 -> [w216]
              tunnel: w192 -> [w212]
              tunnel: [w211] -> w189 mode=indexing
              tunnel: [w210] -> w190 mode=indexing
              tunnel: [w209] -> w191 mode=indexing
              i -> [w213]
              n101 = Multiply(x=w213, y=w212) -> (x*y=w211:dbl)
              n102 = call "FF_BellShapeFun.vi"("Invert(F)"=FALSE, "(r)adius"=w216, "(A)mplitude"=w217, "x"=w211) -> ("y"=w209:dbl)  [unwired: 2 in]
              n103 = call "FF_BellShapeFun.vi"("Invert(F)"=TRUE ("Invert"), "(r)adius"=w218, "(A)mplitude"=w219, "x"=w211) -> ("y"=w210:dbl)  [unwired: 2 in]
            }
            n104 = Bundle(w189, w190) -> (w187:cluster{dbl[], dbl[]})  [unwired: 1 in]
            n105 = Bundle(w189, w191) -> (w188:cluster{dbl[], dbl[]})  [unwired: 1 in]
            n106 = Build Array(w187, w188) -> (→"Normal Force Shape":cluster{dbl[], dbl[]}[])
          }
          event "Leg Property", "Cuff Location", "Extra Wt": Value Change {
            # "in to m"
            # "lb to kg"
            n107 = event-data() -> ()  [unwired: 1 in, 6 out]
            n108 = Unbundle By Name("Cuff Location") -> ("Hip Wd (m)"=w230:dbl, "Hip Ht (m)"=w229:dbl, "Hip Fwd (m)"=w228:dbl, "ThighToKnee"=w227:dbl, "ThighDist (in)"=w226:dbl, "ShankToKnee"=w225:dbl)
            n109 = Unbundle By Name("Leg Property") -> ("Thigh"=w236:dbl, "Shank"=w237:dbl, "Hip"=w238:dbl, "ShankWt"=w239:dbl, "ThighWt"=w240:dbl)
            n110 = Bundle By Name(cluster=T7 {"BodyDim"={"ThighLt (m)"=0.4, "ShankLt (m)"=0.41, "HipWd (m)"=0.32}, "BodyWt"={"Thigh (kg)"=0.0, "Shank (kg)"=0.0}, "Cuff Loc"={"HipCuffWd (m)"=0.4, "HipCuffHt (m)"=0.1, "HipFwdShift (m)"=0.0, "ThighToKnee (m)"=0.25, "ThighCuffDist (m)"=0.0, "ShankToKnee (m)"=0.15}} ("LegProperties"), "BodyDim.ThighLt (m)"=w236, "BodyDim.ShankLt (m)"=w237, "BodyDim.HipWd (m)"=w238, "BodyWt.Thigh (kg)"=w239, "BodyWt.Shank (kg)"=w240) -> (w233:T7)
            n111 = expression code="x*0.0254"(w226) -> (w220:dbl)
            n112 = Bundle By Name(cluster=w233, "Cuff Loc.HipCuffWd (m)"=w230, "Cuff Loc.HipCuffHt (m)"=w229, "Cuff Loc.HipFwdShift (m)"=w228, "Cuff Loc.ThighToKnee (m)"=w227, "Cuff Loc.ThighCuffDist (m)"=w220, "Cuff Loc.ShankToKnee (m)"=w225) -> (w232:T7)
            n113 = call "CAlex2_InitAll.vi"("error in (no error)"=w244, "LegProperties"=w232, "CAlex2 in"=w246) -> ("error out"=w243:errorcluster, "CAlex2 out"=w245:refnum<class "CAlex2_Display.lvclass">)  [unwired: 7 in]
            n114 = expression code="x*0.453592"("Extra Wt") -> (w221:cluster{"Thigh (lb)":dbl, "Shank (lb)":dbl})
            n115 = shared-variable "PXIe-8135\\SharedVariables.lvlib\\LegDim"(w232, error in=w243) -> (error out=w224:errorcluster)
            n116 = shared-variable "PXIe-8135\\SharedVariables.lvlib\\ExtraCuffWt"(w221, error in=w224) -> (error out=w223:errorcluster)
            n117 = shared-variable "PXIe-8135\\SharedVariables.lvlib\\UpdateLeg"(TRUE ("UpdateArm"), error in=w223) -> (error out=w241:errorcluster)
          }
          event "Record Data?": Value Change {
            n118 = event-data() -> ()  [unwired: 1 in, 5 out]
            n119 = shared-variable "PXIe-8135\\SharedVariables.lvlib\\Record?"("Record Data?", error in=w247) -> (error out=w248:errorcluster)
          }
          event "File Name": Value Change {
            n120 = event-data() -> ()  [unwired: 1 in, 6 out]
            n121 = shared-variable "PXIe-8135\\SharedVariables.lvlib\\Record?"(error in=w253) -> (w251:bool, error out=w252:errorcluster)
            n122 = case shown="True" w251 {
              tunnel: [w258 w260] -> w254
              tunnel: w252 -> [w257 w260]
              frame False {
                n123 = shared-variable "PXIe-8135\\SharedVariables.lvlib\\FileName"("File Name", error in=w257) -> (error out=w258:errorcluster)
              }
              frame True {
                n124 = One Button Dialog(message="Filename can not be changed during recording") -> ()  [unwired: 1 in, 1 out]
              }
            }
          }
          event "Motor Mode.Idle", "Motor Mode.Pre", "Motor Mode.PID", "Motor Mode.Pre-Value": Value Change {
            n125 = event-data() -> ("CtlRef"=w267:refnum<vi>)  [unwired: 1 in, 5 out]
            n126 = property class="Ctl"(reference=w267) -> (reference out=w264:refnum<vi>, error out=w265:errorcluster, "Label.Text"=w266:string)  [unwired: 1 in]
            n127 = Close Reference(reference=w264, error in (no error)=w265) -> ()  [unwired: 1 out]
            n128 = case shown="\"Idle\"" w266 {
              tunnel: [ControllerMode."Idle" ("MotorMode") ControllerMode."Idle" ("MotorMode") ControllerMode."FF" ("MotorMode") ControllerMode."PID" ("MotorMode")] -> w268
              tunnel: [w270 w273 w285 w297] -> w262
              tunnel: w261 -> [w270 w272 w284 w297]
              frame Default {
              }
              frame "Idle" {
                n129 = property on="Idle" class="Bool (strict)"("Value"=TRUE, "DisabledEnum"=T9."Disabled" ("Disabled")) -> ()  [unwired: 2 in, 2 out]
                n130 = property on="Pre" class="Bool (strict)"("Value"=FALSE, "DisabledEnum"=T9."Enabled" ("Disabled")) -> ()  [unwired: 2 in, 2 out]
                n131 = property on="PID" class="Bool (strict)"("Value"=FALSE, "DisabledEnum"=T9."Disabled and Grayed Out" ("Disabled")) -> ()  [unwired: 2 in, 2 out]
                n132 = Initialize Array(0.0 ("element"), 8 ("dimension size")) -> (w281:dbl[])
                n133 = shared-variable "PXIe-8135\\SharedVariables.lvlib\\PreTensionValue"(w281, error in=w272) -> (error out=w273:errorcluster)
              }
              frame "Pre" {
                n134 = property on="Idle" class="Bool (strict)"("Value"=FALSE, "DisabledEnum"=T9."Enabled" ("Disabled")) -> ()  [unwired: 2 in, 2 out]
                n135 = property on="Pre" class="Bool (strict)"("Value"=TRUE, "DisabledEnum"=T9."Disabled" ("Disabled")) -> ()  [unwired: 2 in, 2 out]
                n136 = property on="PID" class="Bool (strict)"("Value"=FALSE, "DisabledEnum"=T9."Enabled" ("Disabled")) -> ()  [unwired: 2 in, 2 out]
                n137 = property on="Pre-Value" class="Ring (strict)"() -> ("Value"=w290:u8)  [unwired: 2 in, 2 out]
                n138 = To Double Precision Float(number=w290) -> (double precision float=w289:dbl)
                n139 = Initialize Array(w289, 8 ("dimension size")) -> (w294:dbl[])
                n140 = shared-variable "PXIe-8135\\SharedVariables.lvlib\\PreTensionValue"(w294, error in=w284) -> (error out=w285:errorcluster)
              }
              frame "PID" {
                n141 = property on="Idle" class="Bool (strict)"("Value"=FALSE, "DisabledEnum"=T9."Enabled" ("Disabled")) -> ()  [unwired: 2 in, 2 out]
                n142 = property on="Pre" class="Bool (strict)"("Value"=FALSE, "DisabledEnum"=T9."Disabled and Grayed Out" ("Disabled")) -> ()  [unwired: 2 in, 2 out]
                n143 = property on="PID" class="Bool (strict)"("Value"=TRUE, "DisabledEnum"=T9."Disabled" ("Disabled")) -> ()  [unwired: 2 in, 2 out]
              }
            }
            n144 = shared-variable "PXIe-8135\\SharedVariables.lvlib\\MotorMode"(w268, error in=w262) -> (error out=w263:errorcluster)
          }
          event "CuffWeight", "LegWeight", "Force Field": Value Change {
            n145 = event-data() -> ()  [unwired: 1 in, 6 out]
            n146 = shared-variable "PXIe-8135\\SharedVariables.lvlib\\CompLegWeight"("LegWeight", error in=w305) -> (error out=w308:errorcluster)
            n147 = shared-variable "PXIe-8135\\SharedVariables.lvlib\\CompCuffWeight"("CuffWeight", error in=w308) -> (error out=w307:errorcluster)
            n148 = shared-variable "PXIe-8135\\SharedVariables.lvlib\\GenForceField"("Force Field", error in=w307) -> (error out=w306:errorcluster)
          }
          event "Status 1", "Status 2", "Status 3", "Status 4", "Status 5", "Status 6", "Status 7", "Status 8": Value Change {
            n149 = event-data() -> ()  [unwired: 1 in, 6 out]
            n150 = Build Array("Status 1", "Status 2", "Status 3", "Status 4", "Status 5", "Status 6", "Status 7", "Status 8") -> (w313:bool[])
            n151 = shared-variable "PXIe-8135\\SharedVariables.lvlib\\MotorEnable"(w313, error in=w315) -> (error out=w314:errorcluster)
          }
        }
        n152 = Or(x=w37, y="Stop RT") -> (x .or. y?=w36:bool)
        n153 = call <vilib>:"RemoveWarnings.vi"("error in (no error)"=w37) -> ("error out"=w38:errorcluster)
        n154 = shared-variable "PXIe-8135\\SharedVariables.lvlib\\Stop RT"(w36) -> ()  [unwired: 1 in, 1 out]
        n155 = feedback-in #1(w36) -> ()
        n156 = feedback #1() -> (w40:bool)
      }
      n157 = call <vilib>:"Simple Error Handler.vi"("error in (no error)"=w31) -> ()  [unwired: 4 in, 5 out]
    }
  }
